vi "5_6_matrix_transpose.vi"(3 "n":i32, 4 "m":i32, 5 "A":fxp<+/-,5,6>[](array[numeric])) -> (0 "n":i32, 1 "m":i32, 2 "B":fxp<+/-,5,6>[](array[numeric]))   [LabVIEW 2020]
panel:
  in  "B_type":fxp<+/-,5,6>
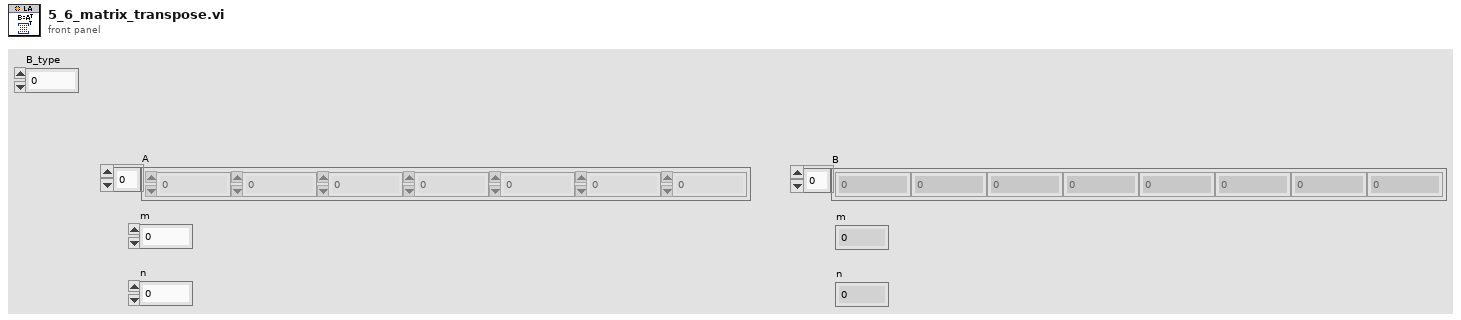
[diagram p1: front panel]
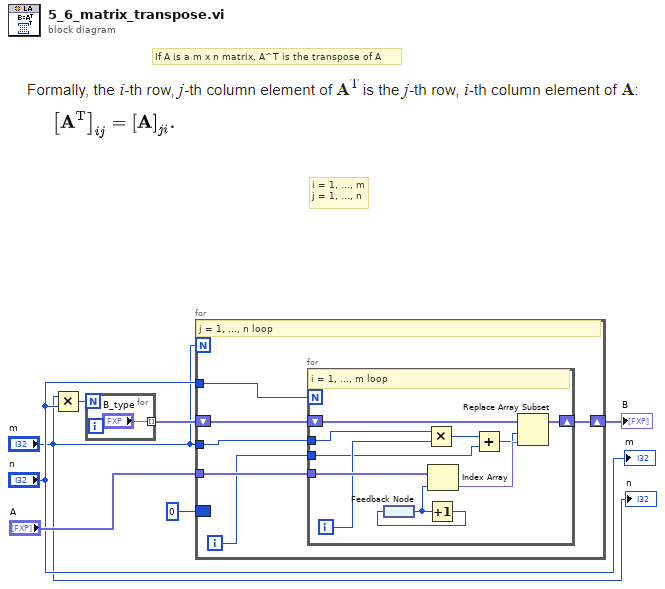
[diagram p0: block diagram]
diagram:
  # "If A is a m x n matrix, A^T is the transpose of A"
  # "i = 1, ..., m\nj = 1, ..., n"
  n1 = Multiply(x="m", y="n") -> (x*y=w4:i32)
  n2 = for {
    N: w4 -> [_]
    tunnel: ["B_type"] -> w5 mode=indexing
  }
  n3 = for {
    N: "m" -> [_]
    tunnel: "A" -> [w14]
    shift-right: [w12] -> w6
    shift-left: w5 -> [w13]
    tunnel: "m" -> [w11]
    tunnel: "n" -> [w9]
    border: 0 -> [_]
    i -> [w10]
    # "j = 1, ..., n loop"
    n4 = for {
      N: w9 -> [_]
      tunnel: w14 -> [w25]
      tunnel: w11 -> [w21]
      tunnel: w10 -> [w19]
      shift-right: [w23] -> w12
      shift-left: w13 -> [w24]
      i -> [w22]
      # "i = 1, ..., m loop"
      n5 = feedback #1() -> (w18:i32)
      n6 = Multiply(x=w21, y=w22) -> (x*y=w20:i32)
      n7 = Increment(x=w18) -> (x+1=w17:i32)
      n8 = feedback-in #1(w17) -> ()
      n9 = Index Array(array=w25, index=w18) -> (element=w16:fxp<+/-,5,6>)
      n10 = Add(x=w20, y=w19) -> (x+y=w15:i32)
      n11 = Replace Array Subset(array=w24, new element=w16, index=w15) -> (w23:fxp<+/-,5,6>[])
    }
  }
  "B" <- w6
  "n" <- "m"
  "m" <- "n"
